vi "Has Connection.vi"(8 "error in (no error)":errorcluster, 11 "Manager in":refnum<class "Manager.lvclass">) -> (0 "error out":errorcluster, 2 "Connected":bool, 3 "Manager out":refnum<class "Manager.lvclass">)   [LabVIEW 2020, in "Stream-Simple-Msg.lvlib" / "Manager.lvclass"]
uses:
  Manager.lvclass
  Manager.lvclass/Manager.ctl
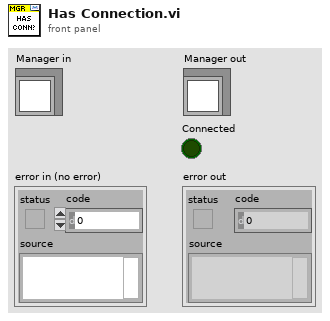
[diagram p1: front panel]
types:
  T1 = typedef "Stream-Simple-Msg.lvlib/Manager.lvclass/Ref Data.ctl" = cluster{"Message Callbacks":map{string, T2[]}, "Endpoints":map{string, T3}, "Stream Endpoints":refnum<class "Endpoint.lvclass">[], "State Callbacks":T5[], "Stream Formats":T4[]}
  T2 = typedef "Stream-Simple-Msg.lvlib/Manager.lvclass/Callback.ctl" = cluster{"VI":refnum<vi>, "Owner":refnum<class>}
  T3 = typedef "Stream-Simple-Msg.lvlib/Manager.lvclass/Mapped Endpoint.ctl" = cluster{"Msg Endpoint":refnum<class "Endpoint.lvclass">, "Format":T4}
  T4 = typedef "Stream-Simple-Msg.lvlib/Format.ctl" = enum16{"LabVIEW Binary", "JSON"}
  T5 = typedef "Stream-Simple-Msg.lvlib/Manager.lvclass/State Callback.ctl" = cluster{"Owner":refnum<class>, "VI":refnum<vi>, "Context":variant}
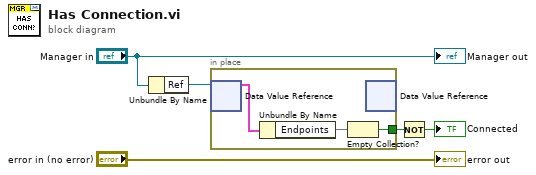
[diagram p0: block diagram]
diagram:
  n1 = Unbundle By Name("Manager in") -> ("Ref"=w4:refnum<data-value>)
  n2 = in-place {
    in-place-border: [w6] -> w2
    n3 = in-place-dvr #1(w4) -> (w8:T1)  [unwired: 1 out]
    n4 = Unbundle By Name(w8) -> ("Endpoints"=w7:map{string, T3})
    n5 = Empty Collection?(1:w7) -> (0:w6:bool)
    n6 = in-place-dvr #1() -> ()  [unwired: 1 in, 2 out]
  }
  n7 = Not(x=w2) -> (.not. x?=→"Connected":bool)
  "error out" <- "error in (no error)"
  "Manager out" <- "Manager in"
